vi "RIO Fusion Multicast Receiver.vi"() -> ()   [LabVIEW 2015]
doc: "Creates a read-only UDP multicast session and receives data on the specified port."
uses:
  <vilib>/Utility/tcp.llb/UDP Multicast Read-Only Open.vi
panel:
  out "error?":bool
  out "Received Data":dbl(graph)
  in  "Stop":bool
  # "Overview: Demonstrates the use of the UDP functions to connect to a UDP multicast session and receive data.\nInstructions:\n1. Ensure UDP Multicast - Sender.vi is already running.\n2. Run the VI.\n3. Click Stop to stop the VI."
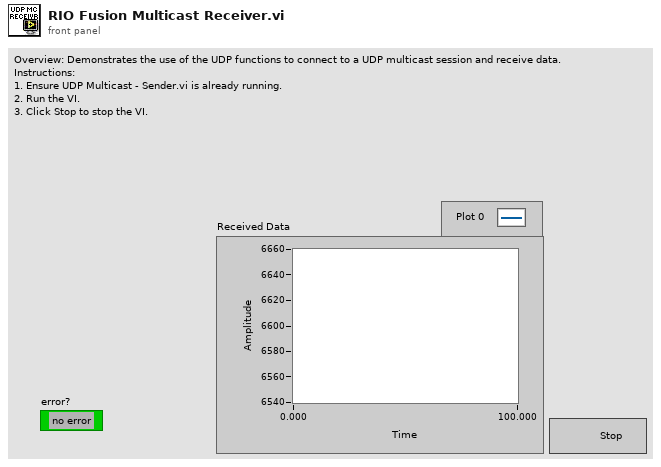
[diagram p1: front panel]
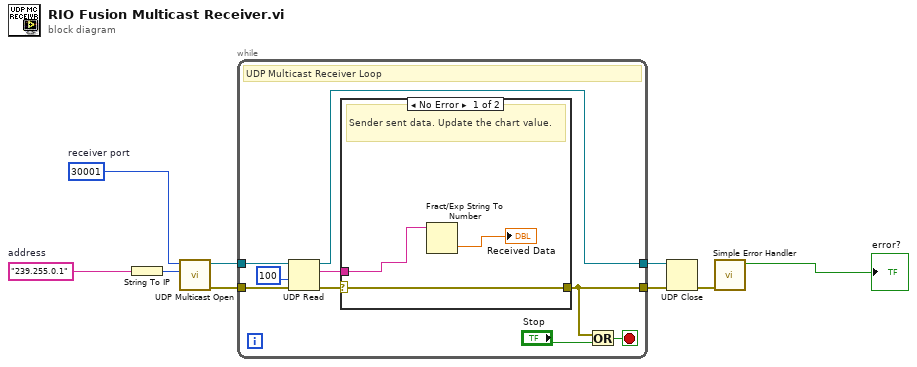
[diagram p0: block diagram]
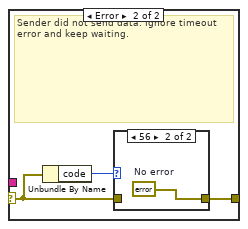
[diagram p2: hidden frame]
diagram:
  w3 = u16 30001  # receiver port
  w8 = "239.255.0.1"  # address
  n1 = String To IP(1:w8) -> (0:w2:u32)
  n2 = call-poly <vilib>:"UDP Multicast Open.vi"("multicast addr"=w2, "port"=w3) -> ("error out"=w5:errorcluster, "connection ID"=w4:refnum<k16>)  [unwired: 7 in, 1 out]
  n3 = while {
    tunnel: w4 -> [w18]
    tunnel: [w10] -> w9
    tunnel: w5 -> [w15]
    tunnel: [w11] -> w6
    stop <- w16 stop-if-true
    # "UDP Multicast Receiver Loop"
    n4 = UDP Read(connection ID=w18, timeout ms (25000)=100, 8:w15) -> (data out=w13:string, error out=w12:errorcluster, 3:w10:refnum<k16>)  [unwired: 3 out]
    n5 = case shown="No Error" w12 {
      selector: w12 -> [w21 w23]
      tunnel: w13 -> [w20 _]
      tunnel: [w21 w22] -> w11
      frame No Error {
        # "Sender sent data. Update the chart value."
        n6 = Fract/Exp String To Number(string=w20) -> (number=→"Received Data":dbl)  [unwired: 3 in, 1 out]
      }
      frame Error {
        # "Sender did not send data. Ignore timeout error and keep waiting."
        n7 = Unbundle By Name(w23) -> ("code"=w24:i32)
        n8 = case shown="56" w24 {
          tunnel: w23 -> [w25 _]
          tunnel: [w25 w26] -> w22
          frame Default {
          }
          frame 56 {
            w26 = errorcluster {"status"=FALSE, "code"=0, "source"=""}  # No error
          }
        }
      }
    }
    n9 = Or(x=w11, y="Stop") -> (x .or. y?=w16:bool)
  }
  n10 = UDP Close(connection ID=w9, 8:w6) -> (error out=w7:errorcluster)  [unwired: 1 out]
  n11 = call <vilib>:"Simple Error Handler.vi"("error in (no error)"=w7) -> ("error?"=→"error?":bool)  [unwired: 1 in, 7 out]
